vi "get_[[]]s.vi"(11 "String":string) -> (3 "Array":string[](array[string]))   [LabVIEW 2022 SP3]
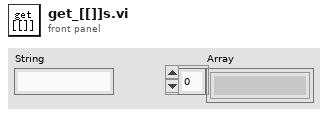
[diagram p1: front panel]
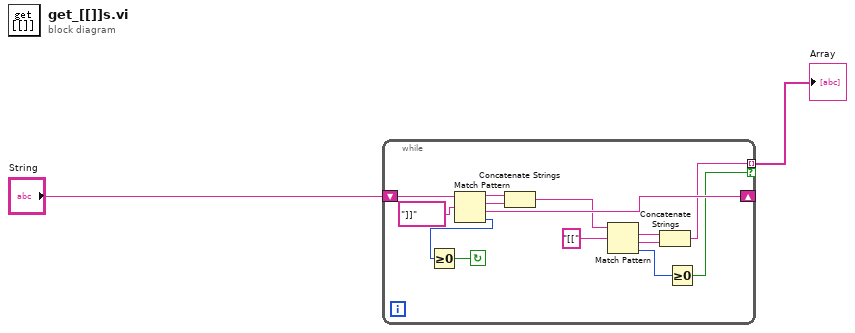
[diagram p0: block diagram]
diagram:
  n1 = while {
    shift-right: [w15] -> _
    shift-left: "String" -> [w16]
    tunnel: [w3] -> w2 mode=indexing if=w10
    stop <- w13 continue-if-true
    n2 = Match Pattern(string=w16, regular expression="]]") -> (before substring=w8:string, match substring=w6:string, after substring=w15:string, offset past match=w12:i32)  [unwired: 1 in]
    n3 = Greater Or Equal To 0?(x=w12) -> (x >= 0?=w13:bool)
    n4 = Concatenate Strings(w8, w6) -> (w7:string)
    n5 = Match Pattern(string=w7, regular expression="[[") -> (match substring=w4:string, after substring=w5:string, offset past match=w11:i32)  [unwired: 1 in, 1 out]
    n6 = Concatenate Strings(w4, w5) -> (w3:string)
    n7 = Greater Or Equal To 0?(x=w11) -> (x >= 0?=w10:bool)
  }
  "Array" <- w2
